vi "SettlingTimeExp.vi"() -> ()   [LabVIEW 2009]
uses:
  <instrlib>/BK Precision 91xx Series/BK Precision 91xx Series.lvlib
panel:
  out "error out":errorcluster
  in  "Serial Configuration":T1={"Parity(0:none)"=0, "Baud Rate (9600)"=9600, "Data Bits(8)"=8, "Flow Control(None)"=0, " Stop Bits(1.0)"=10} {"Stop Bits(1.0)" items=["1.0"=10, "1.5"=15, "2.0"=20]; "Flow Control(None)" items=["None", "XON/XOFF", "RTS/CTS", "XON/XOFF & RTS/CTS", "DTR/DSR", "XON/XOFF & DTR/DSR"]; "Data Bits(8)" items=["7"=7, "8"=8]; "Baud Rate (9600)" items=["2400"=2400, "4800"=4800, "9600"=9600, "19200"=19200, "38400"=38400]; "Parity(0:none)" items=["None", "Odd", "Even", "Mark", "Space"]}
  in  "VISA resource name":refnum<visa-resource-name>
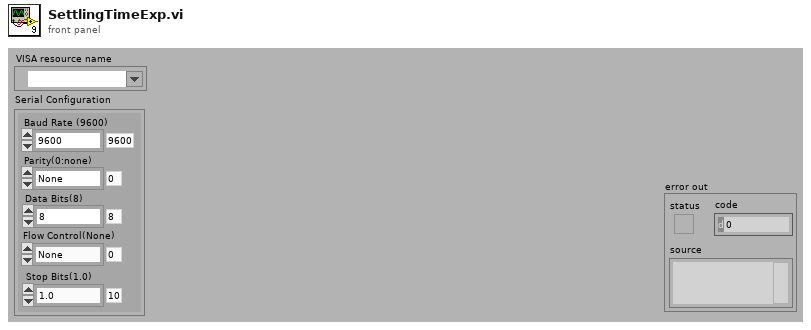
[diagram p1: front panel]
types:
  T1 = cluster{"Parity(0:none)":u16, "Baud Rate (9600)":u16, "Data Bits(8)":u16, "Flow Control(None)":u16, " Stop Bits(1.0)":u16}
  T2 = enum16{"open", "replace", "create", "open or create", "replace or create", "replace or create with confirmation"}
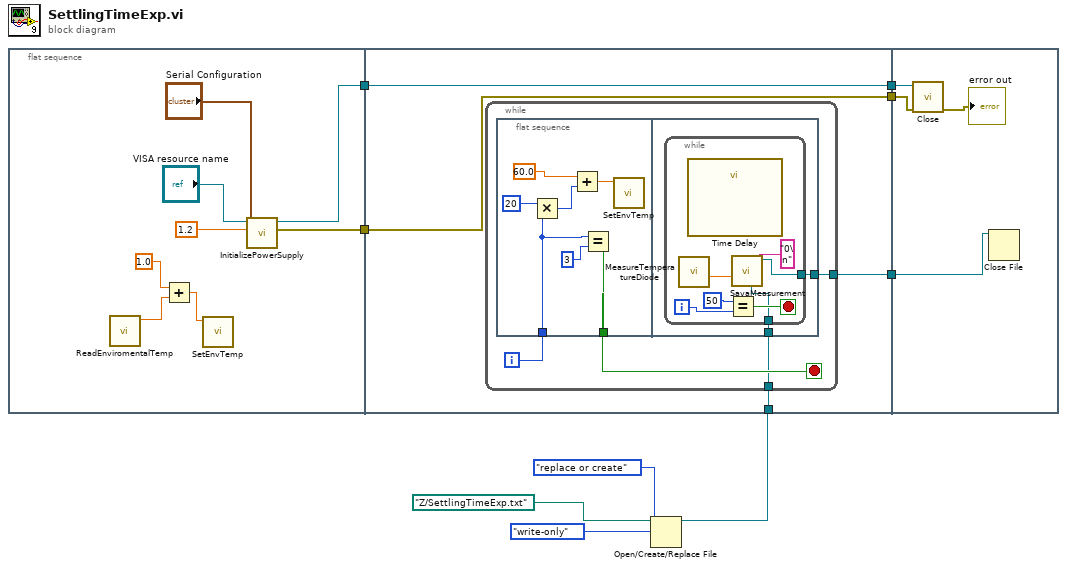
[diagram p0: block diagram]
diagram:
  n1 = flat-sequence {
    tunnel: [w11] -> w6
    tunnel: [w10] -> w3
    tunnel: w6 -> [w21]
    tunnel: [w21] -> w5
    tunnel: [w20] -> w4
    tunnel: w3 -> [w20]
    tunnel: w2 -> [w19]
    tunnel: [w18] -> w1
    tunnel: w5 -> [w44]
    tunnel: w4 -> [w43]
    tunnel: w1 -> [w42]
    frame #0 {
      n2 = call "ReadEnviromentalTemp.vi"() -> ("Probe 1 temperature"=w13:dbl)  [unwired: 10 in, 1 out]
      n3 = Add(x=1.0, y=w13) -> (x+y=w12:dbl)
      n4 = call "SetEnvTemp.vi"("New temperature"=w12) -> ()  [unwired: 10 in, 1 out]
      n5 = call "InitializePowerSupply.vi"("Serial Configuration"="Serial Configuration", "Manual Range(0.00)"=1.2, "VISA resource name"="VISA resource name") -> ("error out"=w10:errorcluster, "VISA resource name out"=w11:refnum<visa-resource-name>)  [unwired: 7 in]
    }
    frame #1 {
      n6 = while {
        tunnel: w19 -> [w23]
        tunnel: [w22] -> w18
        i -> [w25]
        stop <- w24 stop-if-true
        n7 = flat-sequence {
          tunnel: w25 -> [w28]
          tunnel: [w27] -> w24
          tunnel: w23 -> [w34]
          tunnel: [w33] -> w22
          frame #0 {
            n8 = Multiply(x=20, y=w28) -> (x*y=w29:i32)
            n9 = Add(x=60.0, y=w29) -> (x+y=w31:dbl)
            n10 = Equal?(x=w28, y=3) -> (x = y?=w27:bool)
            n11 = call "SetEnvTemp.vi"("New temperature"=w31) -> ()  [unwired: 10 in, 1 out]
          }
          frame #1 {
            n12 = while {
              tunnel: w34 -> [w36]
              tunnel: [w35] -> w33
              i -> [w39]
              stop <- w37 stop-if-true
              n13 = call "MeasureTemperatureDiode.vi"() -> ("Celcius"=w41:dbl)  [unwired: 8 in, 3 out]
              n14 = call "Time Delay"() -> ()  [unwired: 11 in, 1 out]
              n15 = Equal?(x=50, y=w39) -> (x = y?=w37:bool)
              n16 = call "SavaMeasurement.vi"("Measurement"="0\n", "refnum out"=w36, "DiodeTemperature"=w41) -> ("refnum out 2"=w35:refnum<file>)  [unwired: 2 in, 1 out]
            }
          }
        }
      }
    }
    frame #2 {
      n17 = call <instrlib>:"Close.vi"("error in (no error)"=w43, "VISA resource name"=w44) -> ("error out"=→"error out":errorcluster)  [unwired: 9 in]
      n18 = Close File(refnum=w42) -> ()  [unwired: 1 in, 2 out]
    }
  }
  n19 = Open/Create/Replace File(file path (use dialog)=path "Z:/SettlingTimeExp.txt", operation (0:open)=T2."replace or create", access (0:read/write)=enum16{"read/write", "read-only", "write-only"}."write-only") -> (refnum out=w2:refnum<file>)  [unwired: 3 in, 2 out]
